vi "Read States.vi"(8 "error in (no error)":errorcluster, 11 "AttackerBlockTactic in":refnum<class "AttackerBlockTactic.lvclass">) -> (0 "error out":errorcluster, 2 "States":T1, 3 "AttackerBlockTactic out":refnum<class "AttackerBlockTactic.lvclass">)   [LabVIEW 2020, in "AttackerBlockTactic.lvclass"]
uses:
  AttackerBlockTactic.lvclass
  States.ctl
  AttackerBlockTactic.lvclass/AttackerBlockTactic.ctl
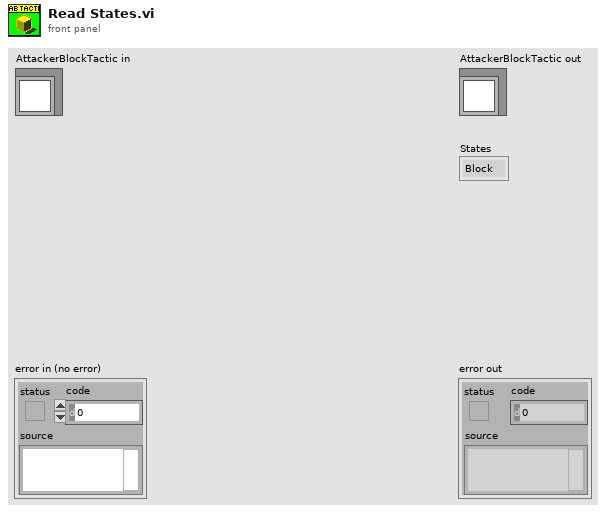
[diagram p1: front panel]
types:
  T1 = typedef "AttackerBlockTactic.lvclass/States.ctl" = enum16{"Block", "Exit"}
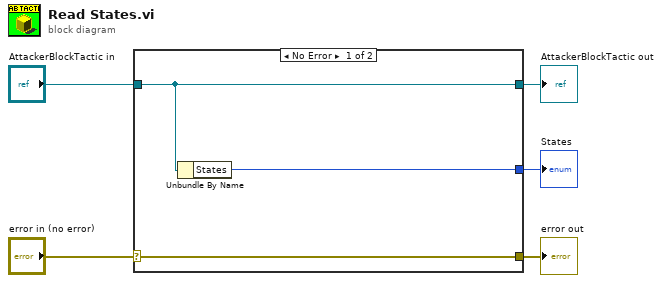
[diagram p0: block diagram]
diagram:
  n1 = case shown="No Error" "error in (no error)" {
    selector: "error in (no error)" -> [w8 w9]
    tunnel: [w8 w9] -> w4
    tunnel: [w7 w10] -> w2
    tunnel: "AttackerBlockTactic in" -> [w7 w10]
    tunnel: [w6 _] -> w1
    frame No Error {
      n2 = Unbundle By Name(w7) -> ("States"=w6:T1)
    }
    frame Error {
    }
  }
  "error out" <- w4
  "AttackerBlockTactic out" <- w2
  "States" <- w1
